vi "Calculate Vertex Array.vi"(8 "error in (no error)":errorcluster, 9 "Coordinates System":enum16{"Cartesian", "Cylindrical", "Spherical"}(ring)=enum."Spherical", 10 "3D Pie Datatype.lvclass in":refnum<class "3D Pie Datatype.lvclass">, 11 "Plot Representation In":T1) -> (0 "error out":errorcluster, 1 "Dup Coordinates System":enum16{"Cartesian", "Cylindrical", "Spherical"}(ring)=enum."Spherical", 2 "3D Pie Datatype.lvclass out":refnum<class "3D Pie Datatype.lvclass">, 3 "Plot Representation Out":T1)   [LabVIEW 2017, in "3D Pie Datatype.lvclass"]
uses:
  <vilib>/Math Plots/3D Math Plots/3D Pie/3D Pie Datatype/3D Pie Datatype.lvclass
  <vilib>/Math Plots/3D Math Plots/3D Plot/3D Plot/Typedef/Plot Representation.ctl
  <vilib>/Math Plots/3D Math Plots/3D Plot/3D Plot/Typedef/Range Clusters.ctl
  <vilib>/Math Plots/3D Math Plots/3D Plot/3D Plot/Typedef/Mesh Data.ctl
  <vilib>/Math Plots/3D Math Plots/3D Pie/3D Pie Datatype/3D Pie Datatype.lvclass/3D Pie Datatype.ctl
  <vilib>/Math Plots/3D Math Plots/3D Plot/3D Plot/3D Plot.lvclass
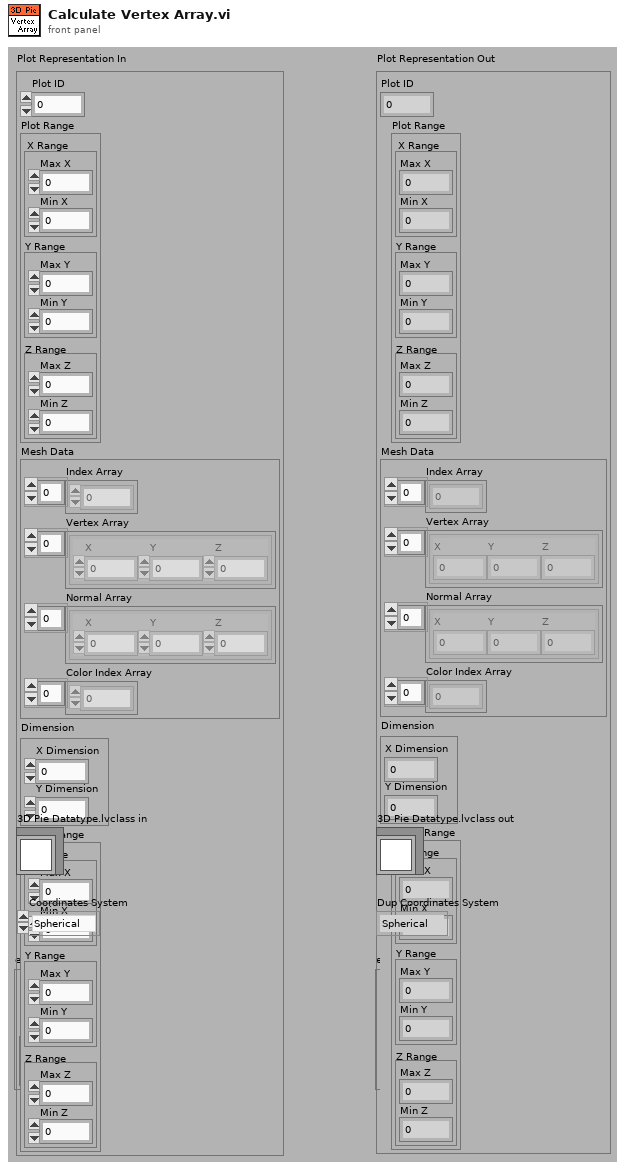
[diagram p1: front panel]
types:
  T1 = typedef "3D Plot.lvclass/Plot Representation.ctl" = cluster{"Plot ID":i32, "Plot Range":T2, "Mesh Data":T3, "Dimension":cluster{"X Dimension":i32, "Y Dimension":i32}, "Ramp Range":T2}
  T2 = typedef "3D Plot.lvclass/Range Clusters.ctl" = cluster{"X Range":cluster{"Max X":sgl, "Min X":sgl}, "Y Range":cluster{"Max Y":sgl, "Min Y":sgl}, "Z Range":cluster{"Max Z":sgl, "Min Z":sgl}}
  T3 = typedef "3D Plot.lvclass/Mesh Data.ctl" = cluster{"Index Array":u32[], "Vertex Array":cluster{"X":sgl, "Y":sgl, "Z":sgl}[], "Normal Array":cluster{"X":sgl, "Y":sgl, "Z":sgl}[], "Color Index Array":i32[]}
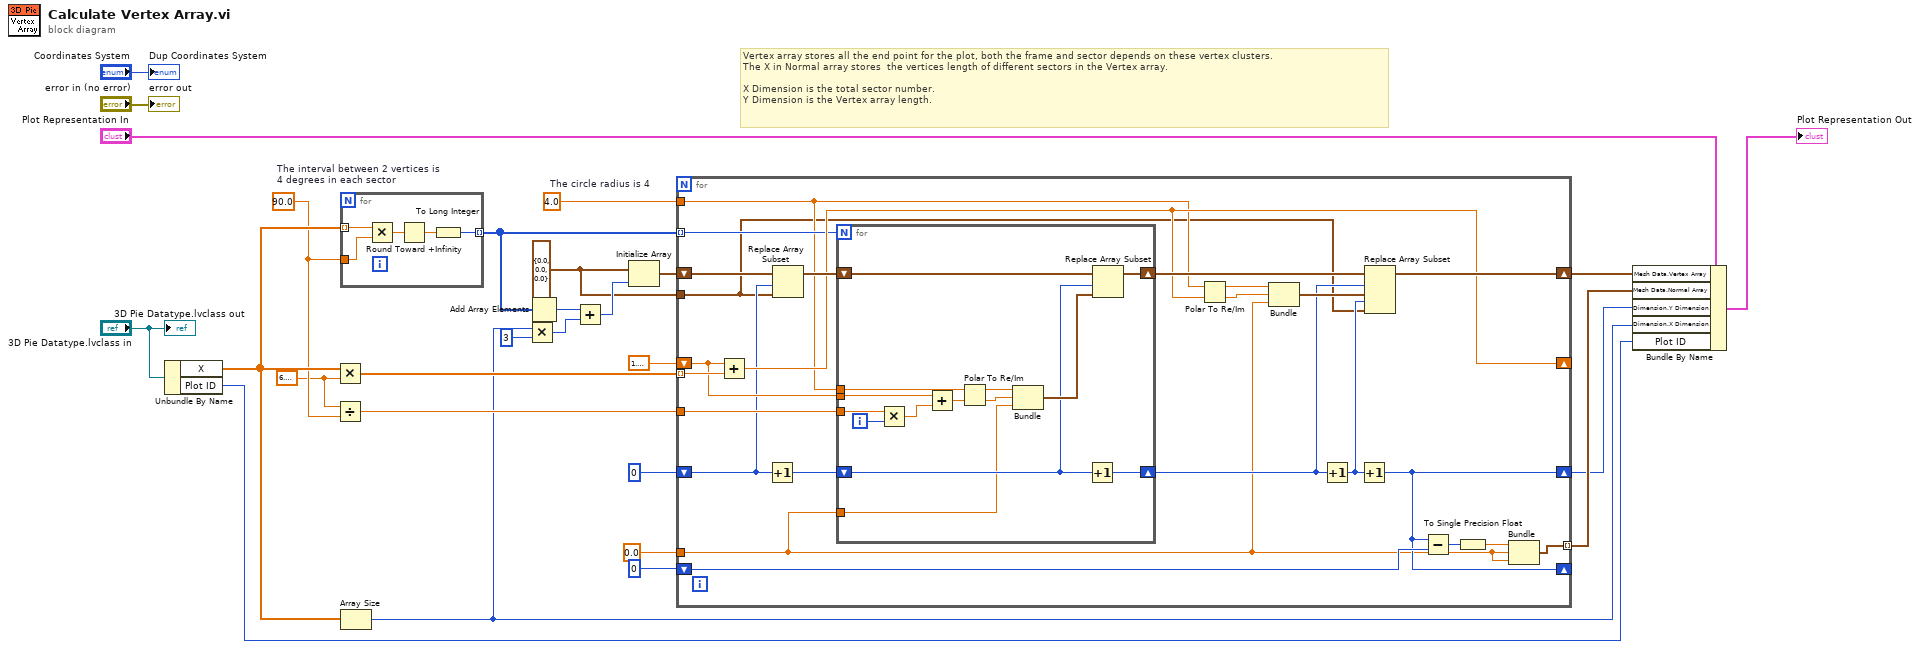
[diagram p0: block diagram]
diagram:
  w1 = sgl 4.0  # The circle radius is 4
  w4 = sgl 90.0  # The interval between 2 vertices is  4 degrees in each sector
  w9 = cluster{sgl, sgl, "Z":sgl} {0.0, 0.0, "Z"=0.0}
  w3 = sgl 6.2831855
  # "Vertex array stores all the end point for the plot, both the frame and sector depends on these vertex clusters.\nThe X in Normal array stores  the vertices length of different sectors in the Vertex array.\n\nX Dimension is the total sector number.\nY Dimension is the Vertex array length."
  n1 = Unbundle By Name("3D Pie Datatype.lvclass in") -> ("X"=w8:sgl[], "Plot ID"=w18:i32)
  n2 = Multiply(x=w8, y=w3) -> (x*y=w10:sgl[])
  n3 = Divide(x=w3, y=w4) -> (x/y=w7:sgl)
  n4 = for {
    tunnel: w8 -> [w32] mode=indexing
    tunnel: w4 -> [w31]
    tunnel: [w28] -> w12 mode=indexing
    n5 = Multiply(x=w32, y=w31) -> (x*y=w30:sgl)
    n6 = Round Toward +Infinity(x=w30) -> (ceil(x): smallest int >= x=w29:sgl)
    n7 = To Long Integer(number=w29) -> (32bit integer=w28:i32)
  }
  n8 = Array Size(array=w8) -> (size(s)=w5:i32)
  n9 = Multiply(x=w5, y=3) -> (x*y=w13:i32)
  n10 = Add Array Elements(numeric array=w12) -> (sum=w16:i32)
  n11 = Add(x=w16, y=w13) -> (x+y=w15:i32)
  n12 = Initialize Array(w9, w15) -> (w17:cluster{sgl, sgl, "Z":sgl}[])
  n13 = for {
    tunnel: w10 -> [w55] mode=indexing
    shift-right: [w50] -> w22
    shift-left: w17 -> [w56]
    tunnel: w7 -> [w53]
    shift-right: [w49] -> _
    shift-left: sgl 1.5707964 -> [w54]
    shift-right: [w38] -> _
    shift-left: 0 -> [w48]
    tunnel: [w36] -> w19 mode=indexing
    tunnel: w12 -> [w44] mode=indexing
    shift-right: [w38] -> w6
    shift-left: 0 -> [w42]
    tunnel: w9 -> [w33]
    tunnel: sgl 0.0 ("Z") -> [w35]
    tunnel: w1 -> [w34]
    n14 = Add(x=w54, y=w55) -> (x+y=w49:sgl)
    n15 = Increment(x=w42) -> (x+1=w43:i32)
    n16 = Replace Array Subset(array=w56, new element=w33, index=w42) -> (w52:cluster{sgl, sgl, "Z":sgl}[])
    n17 = for {
      N: w44 -> [_]
      tunnel: w54 -> [w67]
      tunnel: w53 -> [w69]
      shift-right: [w64] -> w51
      shift-left: w52 -> [w65]
      shift-right: [w61] -> w40
      shift-left: w43 -> [w59]
      tunnel: w35 -> [w58]
      tunnel: w34 -> [w57]
      i -> [w70]
      n18 = Multiply(x=w69, y=w70) -> (x*y=w68:sgl)
      n19 = Add(x=w67, y=w68) -> (x+y=w66:sgl)
      n20 = Polar To Re/Im(2:w66, 3:w57) -> (0:w63:sgl, 1:w62:sgl)
      n21 = Bundle(w62, w63, "Z"=w58) -> (w60:cluster{sgl, sgl, "Z":sgl})  [unwired: 1 out]
      n22 = Increment(x=w59) -> (x+1=w61:i32)
      n23 = Replace Array Subset(array=w65, new element=w60, index=w59) -> (w64:cluster{sgl, sgl, "Z":sgl}[])
    }
    n24 = Polar To Re/Im(2:w49, 3:w34) -> (0:w46:sgl, 1:w45:sgl)
    n25 = Bundle(w45, w46, "Z"=w35) -> (w41:cluster{sgl, sgl, "Z":sgl})  [unwired: 1 out]
    n26 = Increment(x=w40) -> (x+1=w39:i32)
    n27 = Increment(x=w39) -> (x+1=w38:i32)
    n28 = Replace Array Subset(array=w51, new element #1=w41, index #1=w40, new element #2=w33, index #2=w39) -> (w50:cluster{sgl, sgl, "Z":sgl}[])
    n29 = Subtract(x=w38, y=w48) -> (x-y=w47:i32)
    n30 = To Single Precision Float(number=w47) -> (single precision float=w37:sgl)
    n31 = Bundle(w37, "Z"=w35, "Z"=w35) -> (w36:cluster{sgl, "Z":sgl, "Z":sgl})  [unwired: 1 out]
  }
  n32 = Bundle By Name(cluster="Plot Representation In", "Mesh Data.Vertex Array"=w22, "Mesh Data.Normal Array"=w19, "Dimension.Y Dimension"=w6, "Dimension.X Dimension"=w5, "Plot ID"=w18) -> (→"Plot Representation Out":T1)
  "error out" <- "error in (no error)"
  "3D Pie Datatype.lvclass out" <- "3D Pie Datatype.lvclass in"
  "Dup Coordinates System" <- "Coordinates System"
